vi "Read Address.vi"(8 "error in (no error)":errorcluster, 11 "TCP master in":refnum<class "TCP Master.lvclass">) -> (0 "error out":errorcluster, 2 "address":string, 3 "TCP master out":refnum<class "TCP Master.lvclass">)   [LabVIEW 2017, in "SubVIs.lvlib" / "TCP Master.lvclass"]
doc: "Property accessor for the TCP address."
uses:
  <vilib>/Modbus/subvis/Protocol/TCP/TCP Master/TCP Master.lvclass
  <vilib>/Modbus/subvis/Protocol/TCP/TCP Master/TCP Master.lvclass/TCP Master.ctl
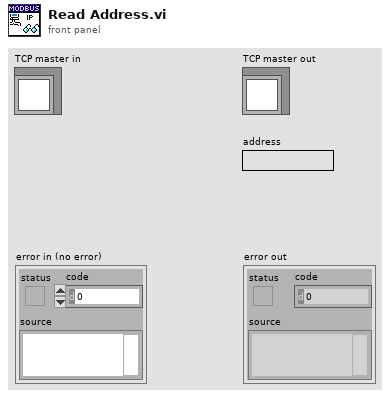
[diagram p1: front panel]
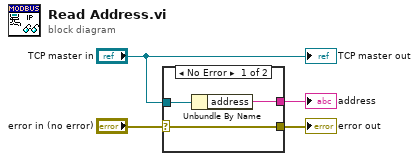
[diagram p0: block diagram]
diagram:
  n1 = case shown="No Error" "error in (no error)" {
    selector: "error in (no error)" -> [w5 w8]
    tunnel: "TCP master in" -> [w7 _]
    tunnel: [w6 _] -> w3
    tunnel: [w5 w8] -> w1
    frame No Error {
      n2 = Unbundle By Name(w7) -> ("address"=w6:string)
    }
    frame Error {
    }
  }
  "error out" <- w1
  "address" <- w3
  "TCP master out" <- "TCP master in"
